vi "Read Discarded.vi"(8 "error in (no error)":errorcluster, 11 "EventDataMessage in":refnum<class "EventDataMessage.lvclass">) -> (0 "error out":errorcluster, 2 "Discarded?":bool, 3 "EventDataMessage out":refnum<class "EventDataMessage.lvclass">)   [LabVIEW 2020, in "ActorEvents.lvlib" / "EventDataMessage.lvclass"]
uses:
  <vilib>/gpm_packages/@cs/mva-viewable/Source/ActorEvents/IEventAggregator Messages/EventDataMessage/EventDataMessage.lvclass
  <vilib>/gpm_packages/@cs/mva-viewable/Source/ActorEvents/IEventAggregator Messages/EventDataMessage/EventDataMessage.lvclass/EventDataMessage.ctl
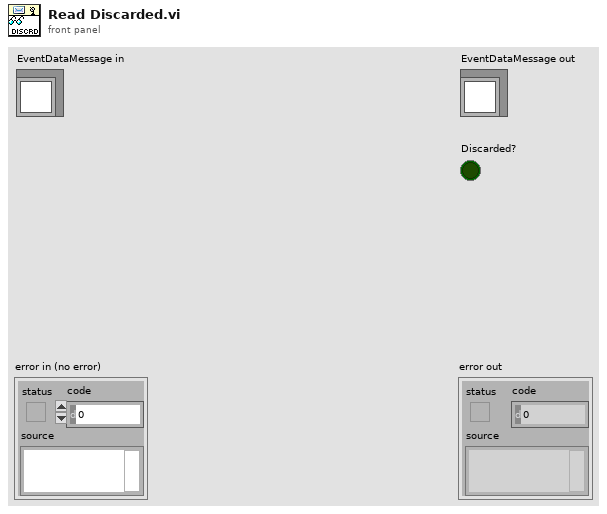
[diagram p1: front panel]
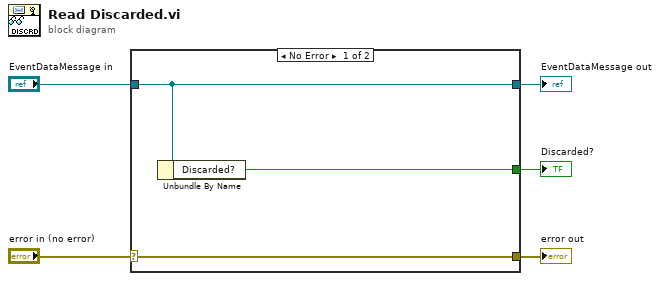
[diagram p0: block diagram]
diagram:
  n1 = case shown="No Error" "error in (no error)" {
    selector: "error in (no error)" -> [w8 w9]
    tunnel: [w8 w9] -> w4
    tunnel: [w7 w10] -> w2
    tunnel: "EventDataMessage in" -> [w7 w10]
    tunnel: [w6 _] -> w1
    frame No Error {
      n2 = Unbundle By Name(w7) -> ("Discarded?"=w6:bool)
    }
    frame Error {
    }
  }
  "error out" <- w4
  "EventDataMessage out" <- w2
  "Discarded?" <- w1
